vi "mono_header.vi"(8 "error in":errorcluster, 11 "connection ID":refnum<k5>) -> (0 "error out":errorcluster, 2 "sensor_sample":T2, 3 "connection ID out":refnum<k5>)   [LabVIEW 2018]
panel:
  in  "byte order (0:big-endian, network order)":T1(ring)=enum."little-endian"
  in  "game_time":u32
  in  "time_stamp":u32
  in  "length":u32
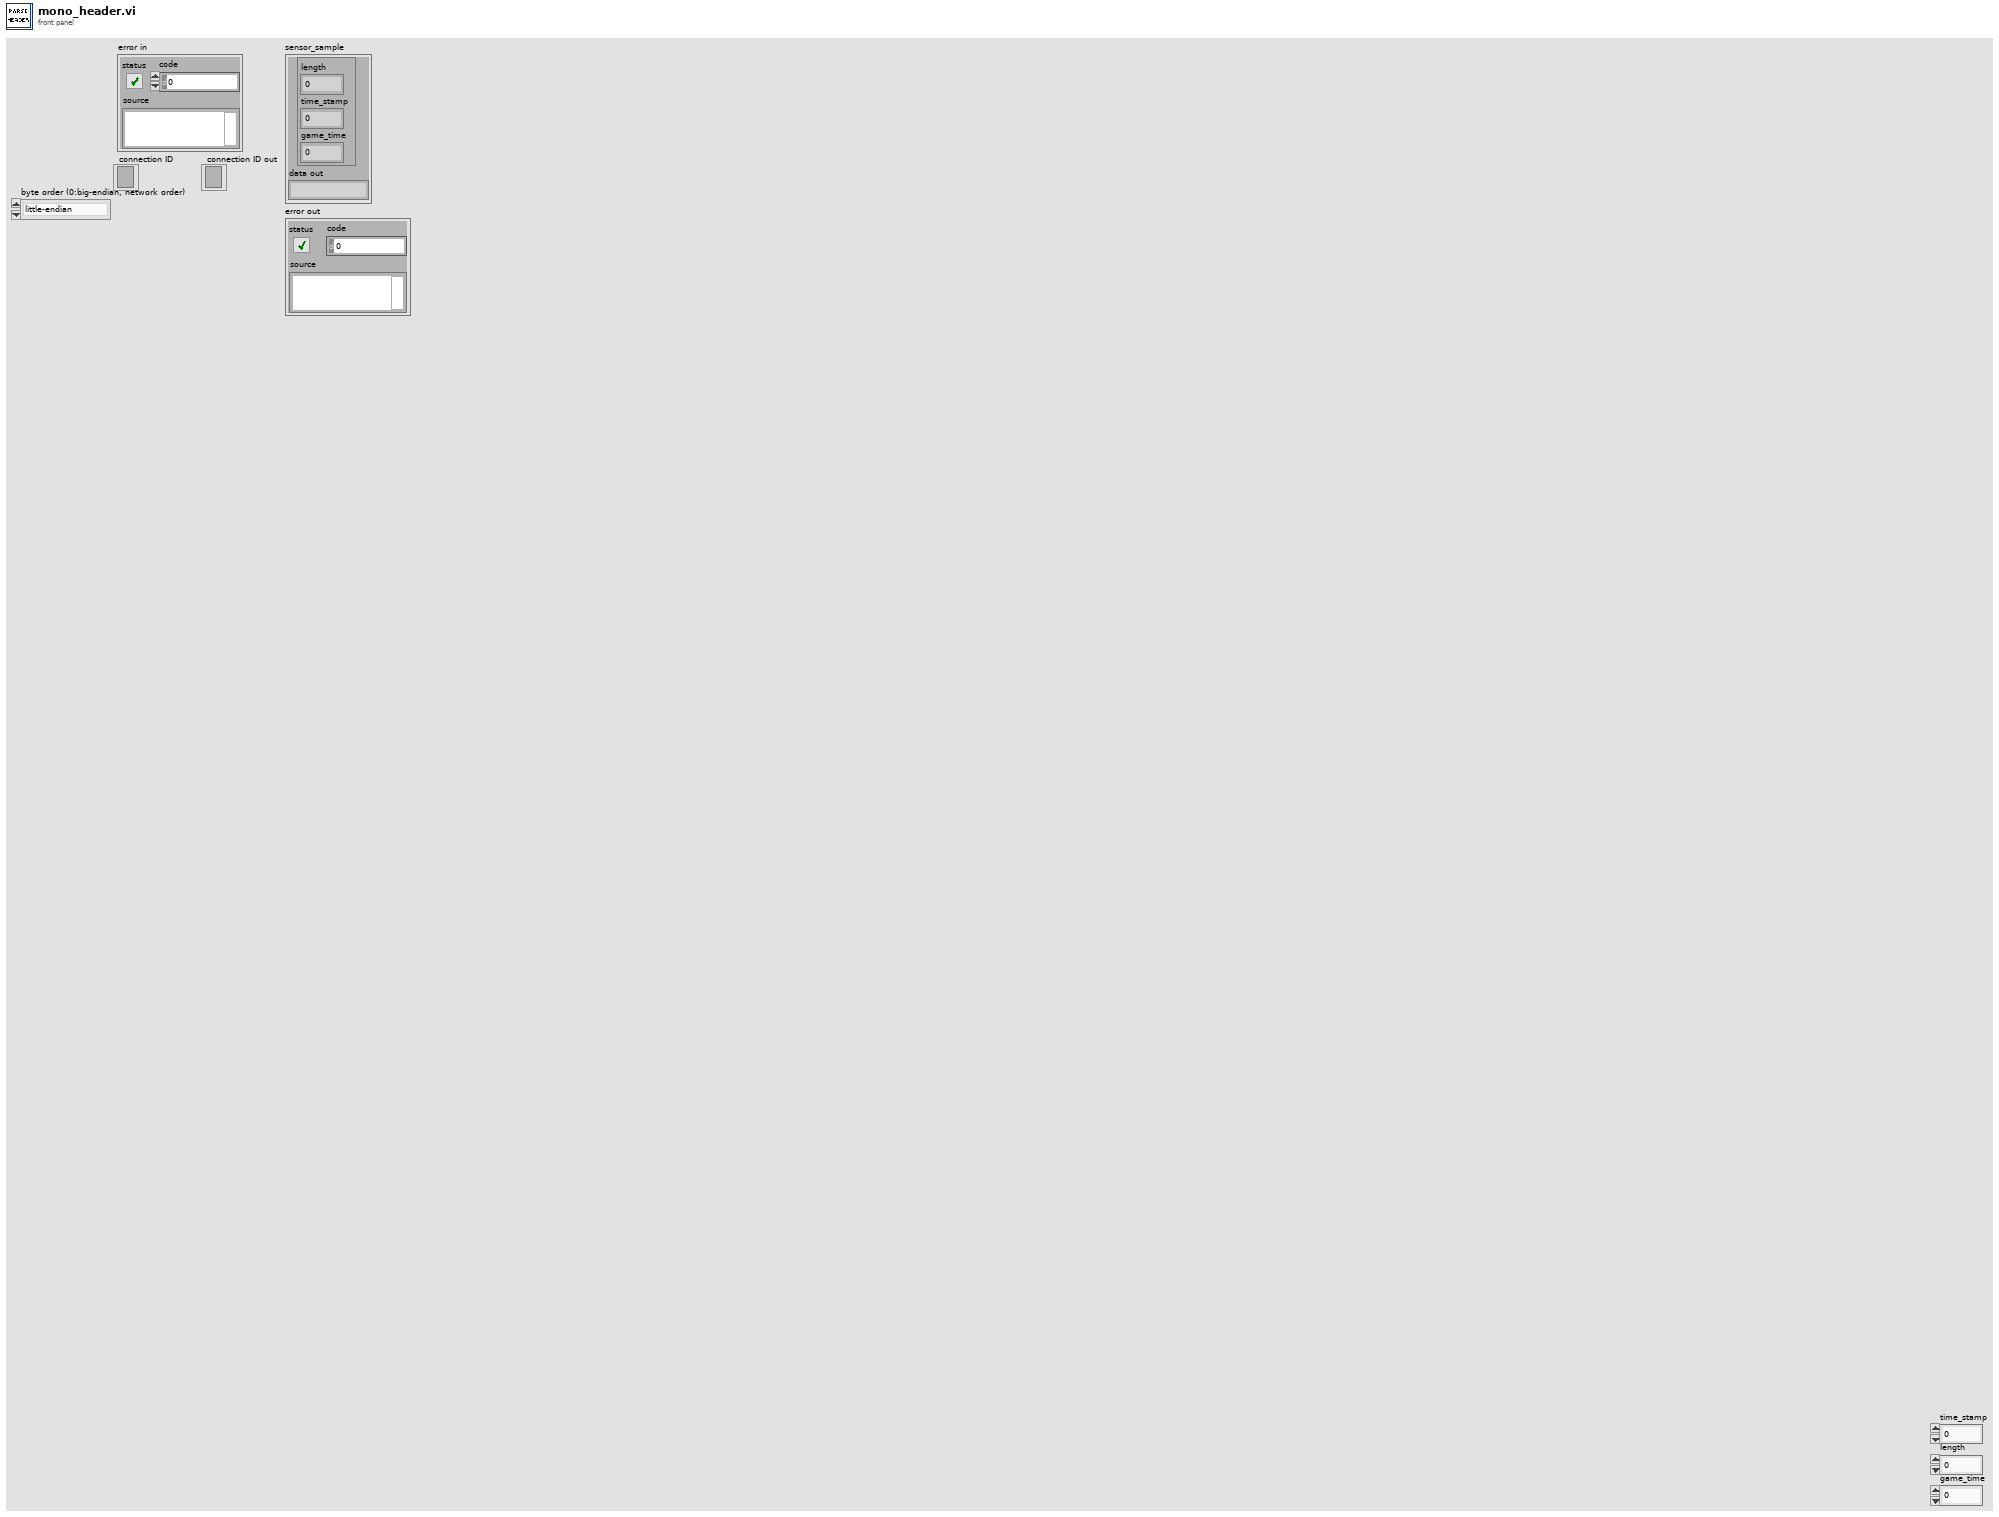
[diagram p1: front panel]
types:
  T1 = enum16{"big-endian, network order", "native, host order", "little-endian"}
  T2 = cluster{cluster{"length":u32, "time_stamp":u32, "game_time":sgl}, "data out":string}
  T3 = cluster{"length":u32, "time_stamp":u32, "game_time":u32}
  T4 = cluster{cluster{"length":u32, "time_stamp":u32, "game_time":u32}, "data out":string}
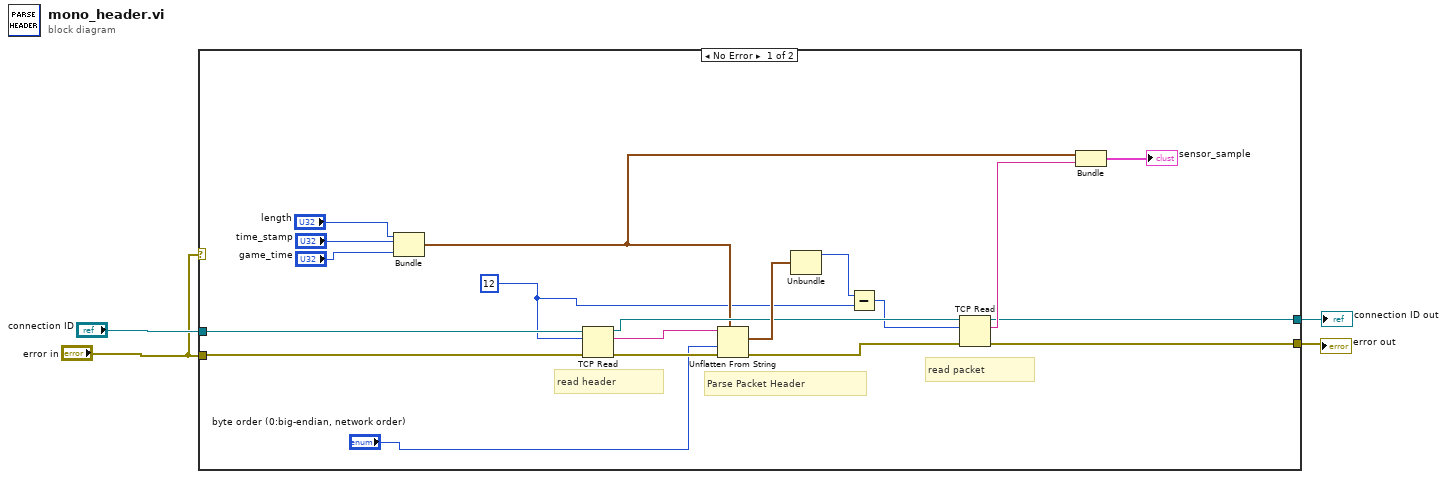
[diagram p0: block diagram]
diagram:
  n1 = case shown="No Error" "error in" {
    tunnel: "error in" -> [w6 w24]
    tunnel: "connection ID" -> [w14 w25]
    tunnel: [w10 w25] -> w3
    tunnel: [w9 w24] -> w2
    frame No Error {
      w7 = 12 ("bytes to read")
      # "read packet"
      # "read header"
      # "Parse Packet Header"
      n2 = Bundle("length"="length", "time_stamp"="time_stamp", "game_time"="game_time") -> (w13:T3)  [unwired: 1 in]
      n3 = TCP Read(connection ID=w14, bytes to read=w7, error in (no error)=w6) -> (connection ID out=w18:refnum<k5>, data out=w19:string, error out=w21:errorcluster)  [unwired: 2 in]
      n4 = Unflatten From String(type=w13, binary string=w19, byte order (0:big-endian, network order)="byte order (0:big-endian, network order)", error in (no error)=w21) -> (value=w20:T3, error out=w22:errorcluster)  [unwired: 1 in, 1 out]
      n5 = Unbundle(w20) -> ("length"=w23:u32)  [unwired: 2 out]
      n6 = Subtract(x=w23, y=w7) -> (x-y=w5:u32)
      n7 = TCP Read(connection ID=w18, bytes to read=w5, error in (no error)=w22) -> (connection ID out=w10:refnum<k5>, data out=w12:string, error out=w9:errorcluster)  [unwired: 2 in]
      n8 = Bundle(w13, "data out"=w12) -> (→"sensor_sample":T4)  [unwired: 1 in]
    }
    frame Error {
    }
  }
  "connection ID out" <- w3
  "error out" <- w2
